vi "和校验Ver1.vi"(1 "输入字符串":u8[](array[numeric])) -> (0 "数值":u8)   [LabVIEW 2015]
panel:
  out "大小":u16
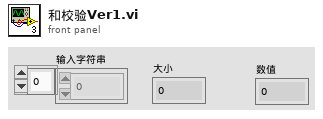
[diagram p1: front panel]
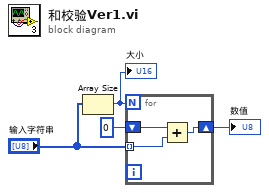
[diagram p0: block diagram]
diagram:
  n1 = Array Size(array="输入字符串") -> (size(s)=w2:i32)
  "大小" <- w2
  n2 = for {
    N: w2 -> [_]
    tunnel: "输入字符串" -> [w5] mode=indexing
    shift-right: [w7] -> w4
    shift-left: u8 0 -> [w6]
    n3 = Add(x=w6, y=w5) -> (x+y=w7:u8)
  }
  "数值" <- w4
